vi "optogeneticsFindNearest.vi"(1 "point":dbl[](array[numeric]), 2 "points":dbl[][](array[numeric])) -> (0 "min index(es)":i32)   [LabVIEW 2017]
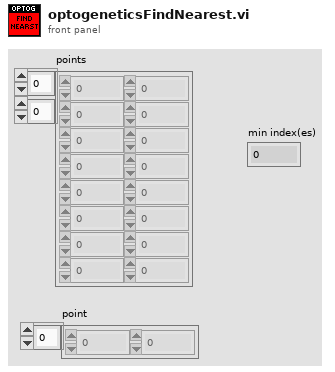
[diagram p1: front panel]
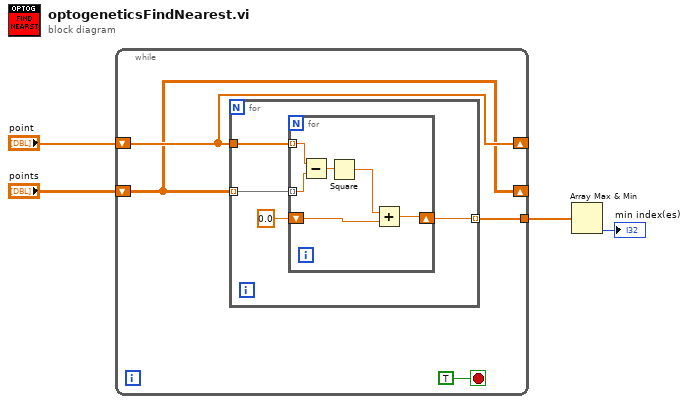
[diagram p0: block diagram]
diagram:
  n1 = while {
    tunnel: [w8] -> w3
    shift-right: [w6] -> _
    shift-left: "point" -> [w6]
    shift-right: [w5] -> _
    shift-left: "points" -> [w5]
    stop <- TRUE stop-if-true
    n2 = for {
      tunnel: w6 -> [w11]
      tunnel: w5 -> [w12] mode=indexing
      tunnel: [w9] -> w8 mode=indexing
      n3 = for {
        tunnel: w12 -> [w17] mode=indexing
        tunnel: w11 -> [w18] mode=indexing
        shift-right: [w13] -> w9
        shift-left: 0.0 -> [w14]
        n4 = Subtract(x=w18, y=w17) -> (x-y=w16:dbl)
        n5 = Square(x=w16) -> (x^2=w15:dbl)
        n6 = Add(x=w15, y=w14) -> (x+y=w13:dbl)
      }
    }
  }
  n7 = Array Max & Min(array=w3) -> (min index (indices)=→"min index(es)":i32)  [unwired: 3 out]
